vi "HexU32 Into String.vi"(8 "Error In":errorcluster, 10 "offset (0)":i32, 11 "Input Data":string="0f 23") -> (0 "Error Out":errorcluster, 2 "Parsed Number Out":string, 3 "Parsed Number Out":u32)   [LabVIEW 2023]
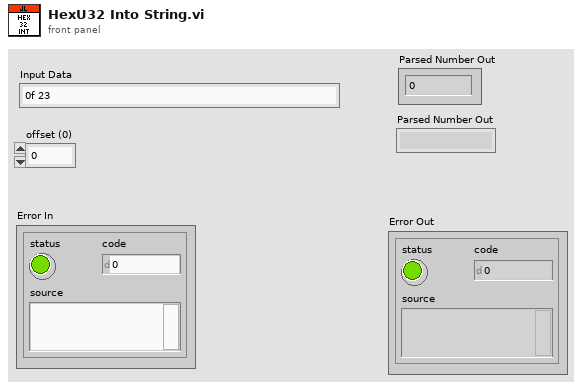
[diagram p1: front panel]
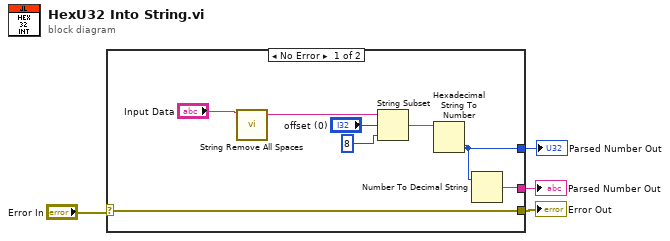
[diagram p0: block diagram]
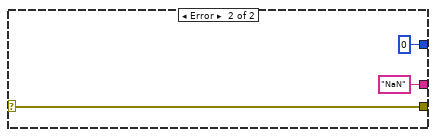
[diagram p2: hidden frame]
diagram:
  n1 = case shown="No Error" "Error In" {
    selector: "Error In" -> [w5 w13]
    tunnel: [w11 "NaN"] -> w4
    tunnel: [w10 u32 0] -> w3
    tunnel: [w5 w13] -> w1
    frame No Error {
      n2 = call "String Remove All Spaces.vi"("Input String"="Input Data") -> ("Spaces Removed"=w7:string)  [unwired: 13 in, 1 out]
      n3 = String Subset(string=w7, offset (0)="offset (0)", length (rest)=8 ("offset (0)")) -> (substring=w6:string)
      n4 = Hexadecimal String To Number(string=w6) -> (number=w10:u32)  [unwired: 2 in, 1 out]
      n5 = Number To Decimal String(number=w10) -> (decimal integer string=w11:string)  [unwired: 1 in]
    }
    frame Error {
    }
  }
  "Parsed Number Out" <- w4
  "Error Out" <- w1
  "Parsed Number Out" <- w3
